vi "Project 6 MHJ.vi"() -> ()   [LabVIEW 2019]
uses:
  <vilib>/Analysis/3filter.llb/Filter Passband Type.ctl
  <vilib>/Analysis/baseanly.llb/Mean (DBL).vi
  <vilib>/Analysis/3filter.llb/Butterworth Filter (DBL).vi
  <vilib>/measure/matone.llb/Extract Single Tone Information 1 Chan.vi
  <vilib>/imath/engines/lvmath2/RunTimeEngine/Managers/WorkSpace/UID Generator.vi
  <vilib>/imath/engines/lvmath2/RunTimeEngine/RunTimeType/NIMS_RunTimeType_From StrictType (excl LVString).vi
  <instcachedir>/0/NIMS_RunTimeType_From StrictType (excl LVString)_D8AFBA86A94845AAA577C895450664BD.lvgen/NIMS_RunTimeType_From StrictType (excl LVString)_D8AFBA86A94845AAA577C895450664BD_000.vi
  <vilib>/imath/engines/lvmath2/RunTimeEngine/LocalVariableDefStatement/MC_LocalVariableDefStatement_Display.vi
  <vilib>/imath/engines/lvmath2/RunTimeEngine/BuiltInFunctions/sin/NIMS_sin(C).vi
  <instcachedir>/0/NIMS_sin(C)_6504C6AC704B4661870B0E93397B11C4.lvgen/NIMS_sin(C)_6504C6AC704B4661870B0E93397B11C4_001.vi
  <vilib>/imath/engines/lvmath2/RunTimeEngine/BuiltInFunctions/cos/NIMS_cos(C).vi
  <instcachedir>/0/NIMS_cos(C)_BED070B05FDB4939A63CB05E18805866.lvgen/NIMS_cos(C)_BED070B05FDB4939A63CB05E18805866_001.vi
  <vilib>/imath/engines/lvmath2/RunTimeEngine/Managers/SymbolTable/Clear UID.vi
  <vilib>/imath/engines/lvmath2/RunTimeEngine/NodeEndStatement/NIMS_NodeEndStatement_Output.vi
  <instcachedir>/0/NIMS_NodeEndStatement_Output_53EC0D466D134D7ABD903AC30B43404B.lvgen/NIMS_NodeEndStatement_Output_53EC0D466D134D7ABD903AC30B43404B_000.vi
  <instcachedir>/0/NIMS_NodeEndStatement_Output_53EC0D466D134D7ABD903AC30B43404B.lvgen/NIMS_NodeEndStatement_Output_53EC0D466D134D7ABD903AC30B43404B_004.vi
  <instcachedir>/0/NIMS_NodeEndStatement_Output_53EC0D466D134D7ABD903AC30B43404B.lvgen/NIMS_NodeEndStatement_Output_53EC0D466D134D7ABD903AC30B43404B_005.vi
  <vilib>/imath/engines/lvmath2/RunTimeEngine/ErrorHandling/NIMS_Finalize Error.vi
  <vilib>/Analysis/NI_AAL_SigProc.lvlib
  <vilib>/Analysis/NI_AALPro.lvlib
  <vilib>/Analysis/NI_AALBase.lvlib
  <vilib>/measure/NI_MAPro.lvlib
  <vilib>/imath/engines/lvmath2/RunTimeEngine/Managers/SymbolTable/NIMS_WorkSpace.lvlib
panel:
  out "concatenated string":string
  out "a(t) string":string
  out "v(t) string":string
  out "x(t) String":string
  in  "Boolean":bool
  out "a(t)":waveform(dbl)(graph)
  out "v(t)":waveform(dbl)(graph)
  out "Raw Data":dynamicdata(graph)
  out "x(t)":waveform(dbl)(graph)
  in  "Amplitude":dbl=1.0
  out "Omega":dbl
  out "detected frequency":dbl format="%.2p"
  in  "stop":bool
  out "damping":dbl
  # "DAQ"
  # "SIM"
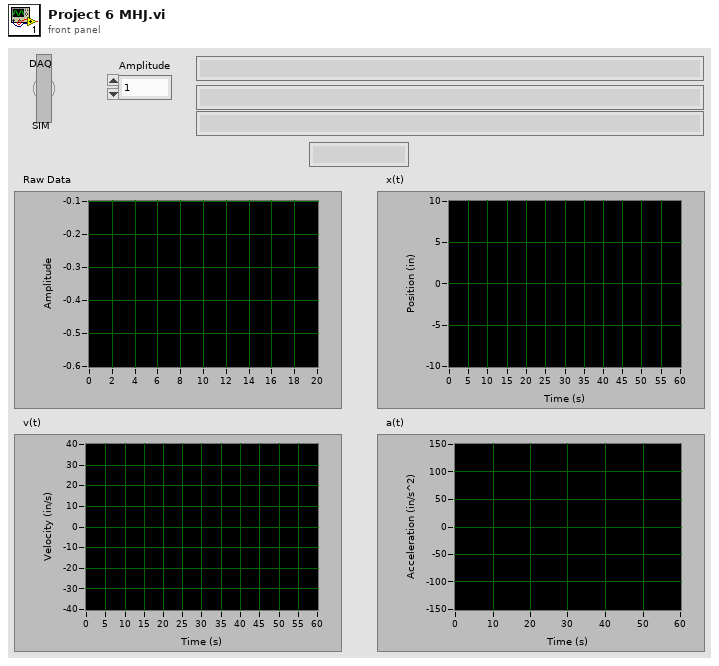
[diagram p1: front panel]
types:
  T1 = typedef "NI_AALBase.lvlib/Filter Passband Type.ctl" = enum32{"Lowpass", "Highpass", "Bandpass", "Bandstop"}
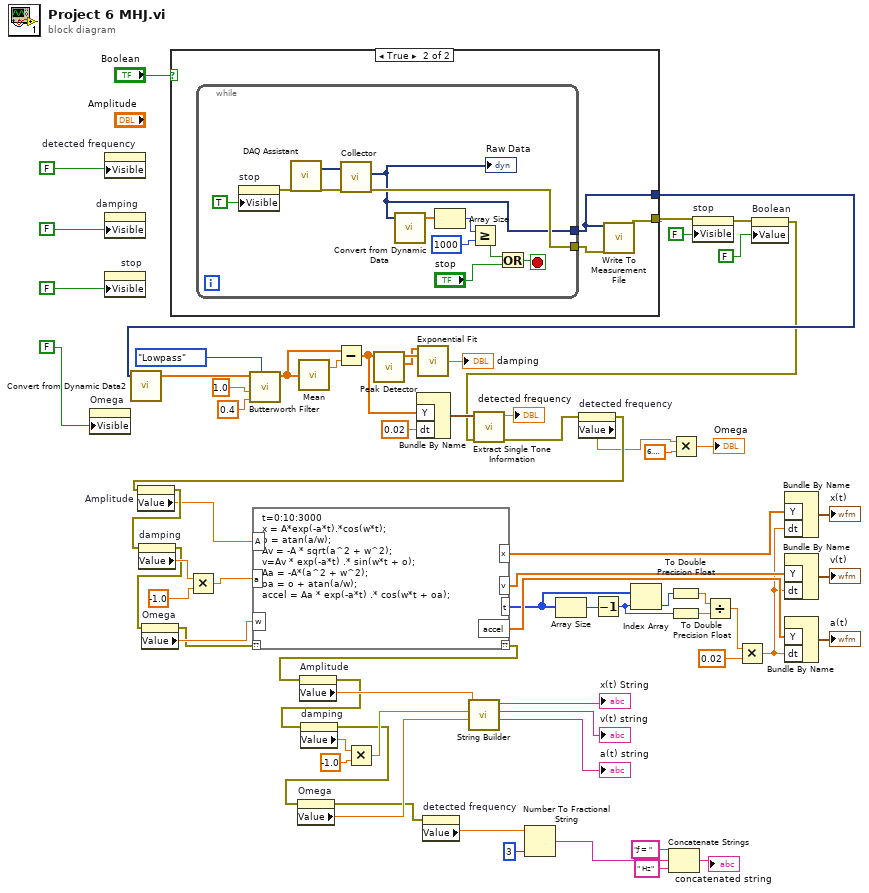
[diagram p0: block diagram]
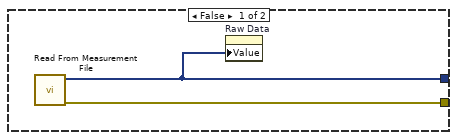
[diagram p2: hidden frame]
diagram:
  n1 = property on="Omega" class="DigNum (strict)"("Visible"=FALSE) -> ()  [unwired: 2 in, 2 out]
  n2 = property on="detected frequency" class="DigNum (strict)"("Visible"=FALSE) -> ()  [unwired: 2 in, 2 out]
  n3 = property on="damping" class="DigNum (strict)"("Visible"=FALSE) -> ()  [unwired: 2 in, 2 out]
  n4 = property on="stop" class="Bool"("Visible"=FALSE) -> ()  [unwired: 2 in, 2 out]
  n5 = case shown="True" "Boolean" {
    tunnel: [w71 w75] -> w27
    tunnel: [w72 w73] -> w33
    frame False {
      n6 = call "Read From Measurement File"() -> ("error out"=w72:errorcluster, "Signals"=w71:dynamicdata)  [unwired: 6 in, 4 out]
      n7 = property on="Raw Data" class="WFGraph (strict)"("Value"=w71) -> ()  [unwired: 2 in, 2 out]
    }
    frame True {
      n8 = while {
        tunnel: [w76] -> w75
        tunnel: [w81] -> w74
        stop <- w84 stop-if-true
        n9 = property on="stop" class="Bool"("Visible"=TRUE) -> (error out=w79:errorcluster)  [unwired: 2 in, 1 out]
        n10 = call "DAQ Assistant"("error in"=w79) -> ("data"=w87:dynamicdata, "error out"=w82:errorcluster)  [unwired: 15 in, 2 out]
        n11 = call "Collector"("error in (no error)"=w82, "Signals"=w87) -> ("error out"=w81:errorcluster, "Collected Signals"=w76:dynamicdata)  [unwired: 8 in]
        "Raw Data" <- w76
        n12 = call "Convert from Dynamic Data"("Dynamic Data Type"=w76) -> ("Array"=w80:dbl[])  [unwired: 3 in]
        n13 = Array Size(array=w80) -> (size(s)=w77:i32)
        n14 = Greater Or Equal?(x=w77, y=1000) -> (x >= y?=w83:bool)
        n15 = Or(x=w83, y="stop") -> (x .or. y?=w84:bool)
      }
      n16 = call "Write To Measurement File"("Signals"=w75, "error in (no error)"=w74) -> ("error out"=w73:errorcluster)  [unwired: 15 in, 2 out]
    }
  }
  n17 = call "Convert from Dynamic Data2"("Dynamic Data Type"=w27) -> ("Array"=w26:dbl[])  [unwired: 3 in]
  n18 = call-poly <vilib>:"Butterworth Filter.vi"("filter type"=Filter_Passband_Type."Lowpass", "low cutoff freq: fl"=0.4, "high cutoff freq: fh"=1.0, "X"=w26) -> ("Filtered X"=w67:dbl[])  [unwired: 4 in, 1 out]
  n19 = call-poly <vilib>:"Mean.vi"("X"=w67) -> ("mean"=w66:dbl)  [unwired: 1 out]
  n20 = Subtract(x=w67, y=w66) -> (x-y=w60:dbl[])
  n21 = call <vilib>:"Peak Detector.vi"("X"=w60) -> ("Amplitudes"=w64:dbl[], "Locations"=w65:dbl[])  [unwired: 6 in, 3 out]
  n22 = Bundle By Name("Y"=w60, "dt"=0.02) -> (w59:waveform(dbl))  [unwired: 1 in]
  n23 = call <vilib>:"Exponential Fit.vi"("Y"=w64, "X"=w65) -> ("damping"=→"damping":dbl)  [unwired: 8 in, 5 out]
  n24 = property on="stop" class="Bool"(error in=w33, "Visible"=FALSE) -> (error out=w24:errorcluster)  [unwired: 1 in, 1 out]
  n25 = property on="Boolean" class="Bool (strict)"(error in=w24, "Value"=FALSE ("Visible")) -> (error out=w23:errorcluster)  [unwired: 1 in, 1 out]
  n26 = call-poly <vilib>:"Extract Single Tone Information.vi"("error in (no error)"=w23, "time signal in"=w59) -> ("error out"=w32:errorcluster, "detected frequency"=→"detected frequency":dbl)  [unwired: 4 in, 4 out]
  n27 = property on="detected frequency" class="DigNum (strict)"(error in=w32) -> (error out=w31:errorcluster, "Value"=w21:dbl)  [unwired: 1 in, 1 out]
  n28 = property on="Amplitude" class="DigNum (strict)"(error in=w31) -> (error out=w57:errorcluster, "Value"=w41:dbl)  [unwired: 1 in, 1 out]
  n29 = property on="damping" class="DigNum (strict)"(error in=w57) -> (error out=w13:errorcluster, "Value"=w62:dbl)  [unwired: 1 in, 1 out]
  n30 = property on="Omega" class="DigNum (strict)"(error in=w13) -> (error out=w12:errorcluster, "Value"=w19:dbl)  [unwired: 1 in, 1 out]
  n31 = Multiply(x=w62, y=-1.0) -> (x*y=w39:dbl)
  n32 = mathscript code="t=0:10:3000\nx = A*exp(-a*t).*cos(w*t);\no = atan(a/w);\nAv = -A * sqrt(a^2 + w^2);\nv=Av * exp(-a*t) .* sin(w*t + o);\nAa = -A*(a^2 + w^2);\noa = o + atan(a/w);\naccel = Aa * exp(-a*t) .* cos(w*t + oa);"("??"=w12, "A"=w41, "a"=w39, "w"=w19) -> ("??"=w11:errorcluster, "x"=w56:dbl[], "v"=w52:cdb[], "t"=w46:i32[], "accel"=w51:cdb[])
  n33 = property on="Amplitude" class="DigNum (strict)"(error in=w11) -> (error out=w10:errorcluster, "Value"=w18:dbl)  [unwired: 1 in, 1 out]
  n34 = property on="damping" class="DigNum (strict)"(error in=w10) -> (error out=w9:errorcluster, "Value"=w16:dbl)  [unwired: 1 in, 1 out]
  n35 = property on="Omega" class="DigNum (strict)"(error in=w9) -> (error out=w2:errorcluster, "Value"=w14:dbl)  [unwired: 1 in, 1 out]
  n36 = Multiply(x=w16, y=-1.0) -> (x*y=w15:dbl)
  n37 = property on="detected frequency" class="DigNum (strict)"(error in=w2) -> ("Value"=w1:dbl)  [unwired: 1 in, 2 out]
  n38 = call "String Builder.vi"("Omega"=w14, "damping"=w15, "A"=w18) -> ("a(t) string"=→"a(t) string":string, "v(t) string"=→"v(t) string":string, "x(t) string"=→"x(t) String":string)  [unwired: 6 in]
  n39 = Number To Fractional String(number=w1, precision (6)=i16 3) -> (F-format string=w6:string)  [unwired: 2 in]
  n40 = Array Size(array=w46) -> (size(s)=w48:i32)
  n41 = Decrement(x=w48) -> (x-1=w45:i32)
  n42 = Index Array(array=w46, index=w45) -> (element=w47:i32)
  n43 = Concatenate Strings("ƒ = " ("string"), w6, " Hz" ("string")) -> (→"concatenated string":string)
  n44 = Multiply(x=w21, y=6.283185307179586) -> (x*y=→"Omega":dbl)
  n45 = To Double Precision Float(number=w47) -> (double precision float=w36:dbl)
  n46 = To Double Precision Float(number=w45) -> (double precision float=w42:dbl)
  n47 = Divide(x=w36, y=w42) -> (x/y=w44:dbl)
  n48 = Multiply(x=w44, y=0.02) -> (x*y=w43:dbl)
  n49 = Bundle By Name("Y"=w56, "dt"=w43) -> (→"x(t)":waveform(dbl))  [unwired: 1 in]
  n50 = Bundle By Name("Y"=w52, "dt"=w43) -> (→"v(t)":waveform(cdb))  [unwired: 1 in]
  n51 = Bundle By Name("Y"=w51, "dt"=w43) -> (→"a(t)":waveform(cdb))  [unwired: 1 in]
